vi "Search String Bi-Directional.vi"(0 "Input String":string, 1 "Ignore Case?":bool, 5 "Search String":string, 7 "Selection End":u32, 9 "Selection Start":u32, 11 "Direction":enum32{"reverse", "forward"}(ring)=enum."forward") -> (10 "Offset in String":i32)   [LabVIEW 2014]
doc: "Searches a string in either forward or backward direction."
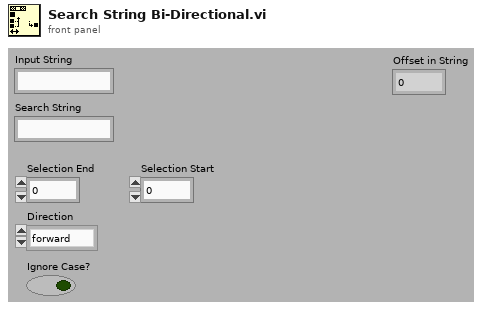
[diagram p1: front panel]
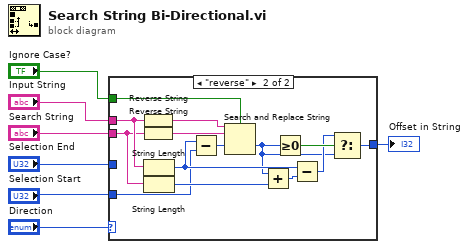
[diagram p0: block diagram]
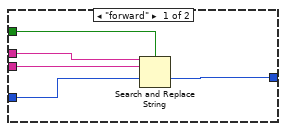
[diagram p2: hidden frame]
diagram:
  n1 = case shown="\"reverse\"" "Direction" {
    tunnel: "Search String" -> [w12 w19]
    tunnel: "Input String" -> [w11 w22]
    tunnel: "Selection End" -> [w10 _]
    tunnel: "Ignore Case?" -> [w9 w26]
    tunnel: "Selection Start" -> [_ w17]
    tunnel: [w8 w13] -> w1
    frame "forward" {
      n2 = Search and Replace String(case sensitive?=w9, input string=w11, search string=w12, offset=w10) -> (offset past replacement=w8:i32)  [unwired: 1 in, 6 out]
    }
    frame "reverse" {
      n3 = Reverse String(1:w22) -> (0:w25:string)
      n4 = Reverse String(1:w19) -> (0:w20:string)
      n5 = String Length(string=w22) -> (length=w23:i32)
      n6 = String Length(string=w19) -> (length=w18:i32)
      n7 = Subtract(x=w23, y=w17) -> (x-y=w24:u32)
      n8 = Search and Replace String(case sensitive?=w26, input string=w25, search string=w20, offset=w24) -> (offset past replacement=w14:i32)  [unwired: 1 in, 6 out]
      n9 = Add(x=w14, y=w18) -> (x+y=w21:i32)
      n10 = Greater Or Equal To 0?(x=w14) -> (x >= 0?=w16:bool)
      n11 = Subtract(x=w23, y=w21) -> (x-y=w15:i32)
      n12 = Select(t=w15, s=w16, f=w14) -> (s? t:f=w13:i32)
    }
  }
  "Offset in String" <- w1
